vi "burn_warn_subVI.vi"(11 "Placeholder\nSfc Temp":dbl) -> (2 "Numeric":dbl, 3 "String":string)   [LabVIEW 2021]
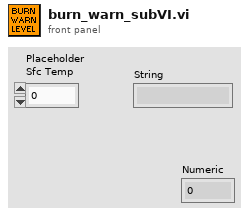
[diagram p1: front panel]
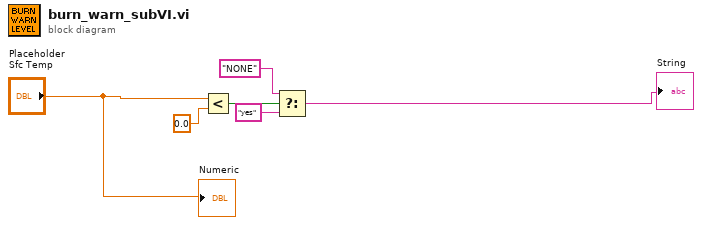
[diagram p0: block diagram]
diagram:
  n1 = Less?(x="Placeholder\nSfc Temp", y=0.0) -> (x < y?=w4:bool)
  n2 = Select(t="NONE", s=w4, f="yes") -> (s? t:f=→"String":string)
  "Numeric" <- "Placeholder\nSfc Temp"
